vi "ReadRangeFileSubVI.vi"(11 "Input Path":path) -> (1 "array type (2D Dbl) 2":dbl[][](array[numeric]), 2 "Output Array":dbl[][](array[numeric]), 3 "String":string, 4 "array type (2D Dbl)":dbl[](array[numeric]), 5 "Searched Part of 2D Array":dbl[](array[numeric]))   [LabVIEW 2019]
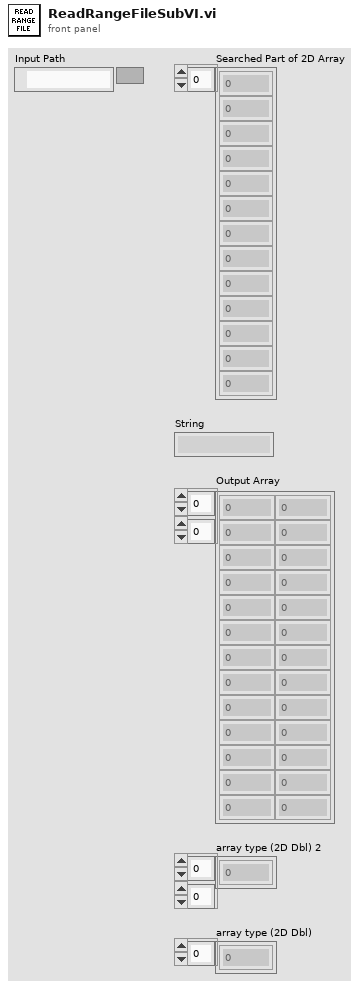
[diagram p1: front panel]
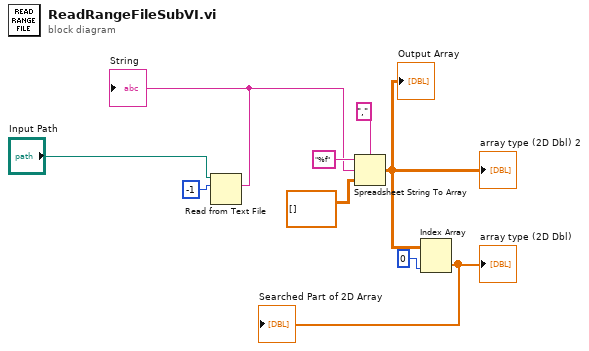
[diagram p0: block diagram]
diagram:
  n1 = Read from Text File(file (use dialog)="Input Path", count=-1) -> (text=w3:string)  [unwired: 2 in, 3 out]
  "String" <- w3
  n2 = Spreadsheet String To Array(delimiter (Tab)=",", format string="%f", spreadsheet string=w3, array type (2D Dbl)=dbl[][] []) -> (array=w1:dbl[][])
  "Output Array" <- w1
  "array type (2D Dbl) 2" <- w1
  n3 = Index Array(array=w1, index (col)=0 ("disabled index (col)")) -> (element=→"Searched Part of 2D Array" →"array type (2D Dbl)":dbl[])  [unwired: 1 in]
